vi "Dequeue Data from RxFIFO (Node).vi"(7 "Timeout":i32, 8 "error in":errorcluster, 9 "Input Valid":bool=TRUE, 11 "FIFOs: I/O Node":T1) -> (0 "error out":errorcluster, 1 "Received Data Valid":bool, 2 "Received Data":u64, 3 "FIFOs: I/O Node":T1)   [LabVIEW 2014, in "IO Node Logic Template.lvlib"]
uses:
  IO Node Logic Template.lvlib
  Controls/NodeResources FIFOs.ctl
  <vilib>/rvi/DataTransferAndStorage/Container/Common/niFpgaContainerExecOnDevCompGetState.vi
  <vilib>/rvi/Emulation/niFpgaEmulationIsFPGAContextNoSignature.vi
  <vilib>/rvi/Emulation/niFpgaSctlEmulationGetInTimedLoop.vi
  <vilib>/rvi/errors/niFpgaSetErrorForExecOnDevCompSimple.vi
  <vilib>/rvi/eio/common/nirviEmuReportErrorAndStop.vi
  <vilib>/rvi/DataTransferAndStorage/Container/Common/niFpgaContainerGetUniqueNameForEmu.vi
  <vilib>/rvi/FIFO/Fifo_Resource/nirvififoEmulationSetSize.vi
  <vilib>/rvi/FIFO/Fifo_Resource/nirviFifoEmulationQueueMgr.vi
  <instcachedir>/0/nirviFifoEmulationQueueMgr_E5CAEC123FF24DC58D834DCA3CDAA9B5.lvgen/nirviFifoEmulationQueueMgr_E5CAEC123FF24DC58D834DCA3CDAA9B5_005.vi
  <vilib>/rvi/FIFO/Fifo_Resource/nirvififoEmulationDetermineInputValidOut.vi
  <vilib>/rvi/FIFO/Fifo_Resource/nirvififoEmulationCreateLock.vi
  <vilib>/rvi/Emulation/niFpgaProcessEmulError.vi
  <vilib>/rvi/FIFO/Fifo_Resource/nirvififoEmulationObtainLock.vi
  <vilib>/rvi/FIFO/Fifo_Resource/nirvififoEmulationReleaseLock.vi
  <vilib>/rvi/occurrence/nirviWaitOnOccurrenceBase.vi
  <vilib>/rvi/errors/nirviReportUnexpectedCaseInternalError.vi
  <vilib>/rvi/errors/nirviReportUnexpectedCaseInternalError (U32).vi
  <vilib>/rvi/interface/RandomDataEmulation/niFpgaRandomDataHandleErrors.vi
  <vilib>/rvi/DataTransferAndStorage/Container/XNode/niFpgaContainer.xnode
  <vilib>/rvi/FIFO/Fifo_Resource/niFpgaFifoEmulationRefIn.vi
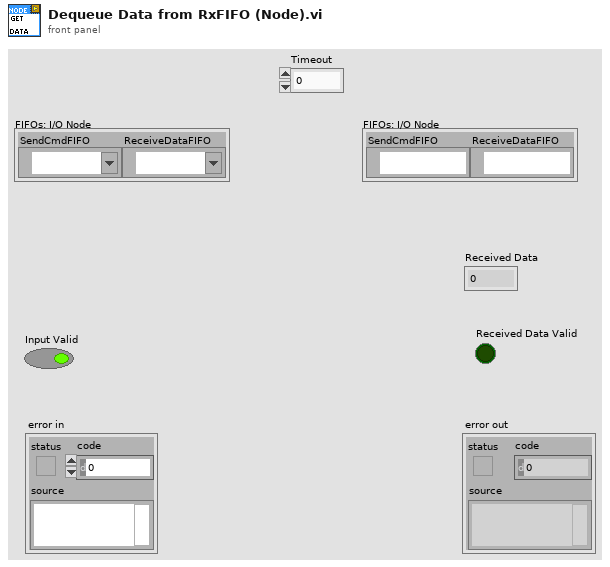
[diagram p1: front panel]
types:
  T1 = typedef "IO Node Logic Template.lvlib/NodeResources FIFOs.ctl" = cluster{"SendCmdFIFO":refnum<k21>, "ReceiveDataFIFO":refnum<k21>}
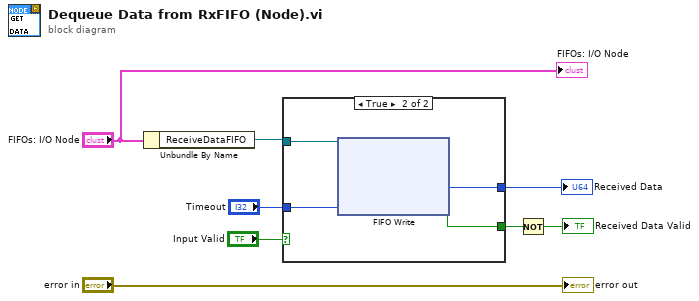
[diagram p0: block diagram]
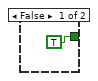
[diagram p2: hidden frame]
diagram:
  n1 = Unbundle By Name("FIFOs: I/O Node") -> ("ReceiveDataFIFO"=w4:refnum<k21>)
  n2 = case shown="True" "Input Valid" {
    tunnel: [TRUE ("Timed Out?") w13] -> w6
    tunnel: w4 -> [_ w12]
    tunnel: "Timeout" -> [_ w11]
    tunnel: [_ w10] -> w1
    frame False {
    }
    frame True {
      n3 = xnode "FIFO Write"("Timeout"=w11, "FIFO In"=w12) -> ("Element"=w10:u64, "Timed Out?"=w13:bool)  [unwired: 1 out]
    }
  }
  "Received Data" <- w1
  n4 = Not(x=w6) -> (.not. x?=→"Received Data Valid":bool)
  "error out" <- "error in"
  "FIFOs: I/O Node" <- "FIFOs: I/O Node"
